vi "A to B(n points).vi"(1 "N":u8, 2 "B":dbl[](array[numeric]), 3 "A":dbl[](array[numeric])) -> (0 "R":dbl[][](array[numeric]))   [LabVIEW 2017]
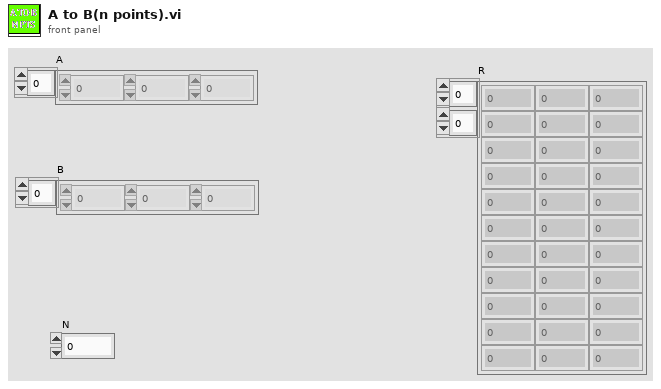
[diagram p1: front panel]
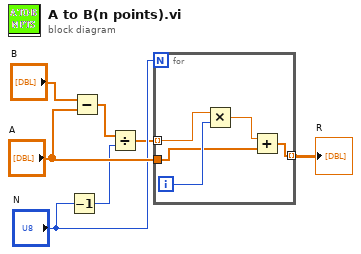
[diagram p0: block diagram]
diagram:
  n1 = Decrement(x="N") -> (x-1=w4:u8)
  n2 = Subtract(x="B", y="A") -> (x-y=w3:dbl[])
  n3 = Divide(x=w3, y=w4) -> (x/y=w2:dbl[])
  n4 = for {
    N: "N" -> [_]
    tunnel: "A" -> [w9]
    tunnel: w2 -> [w12] mode=indexing
    tunnel: [w8] -> w1 mode=indexing
    i -> [w11]
    n5 = Multiply(x=w12, y=w11) -> (x*y=w10:dbl)
    n6 = Add(x=w10, y=w9) -> (x+y=w8:dbl[])
  }
  "R" <- w1
